vi "GarageDoorOpenCommand_Create.vi"(8 "error in":errorcluster, 10 "GarageDoor":refnum<class "GarageDoor.lvclass">, 11 "reference in":refnum<class "GarageDoorOpenCommand.lvclass">) -> (0 "error out":errorcluster, 3 "reference out":refnum<class "GarageDoorOpenCommand.lvclass">)   [LabVIEW 2020, in "GarageDoorOpenCommand.lvclass"]
uses:
  GarageDoorOpenCommand.lvclass
  C:/Projects/OpenGDS_DesignPatterns/Command1/Command_class/Command.lvclass
  GarageDoor_class/GarageDoor.lvclass
  Command_class/Command.lvclass
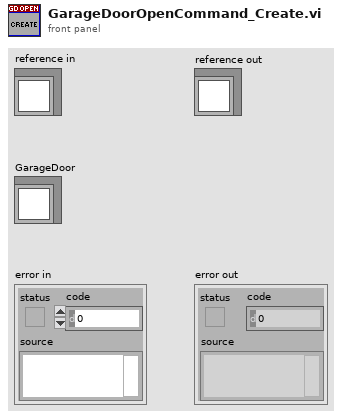
[diagram p1: front panel]
types:
  T1 = typedef "GarageDoorOpenCommand.lvclass/ObjectAttributes.ctl" = cluster{"GarageDoor":refnum<class "GarageDoor.lvclass">}
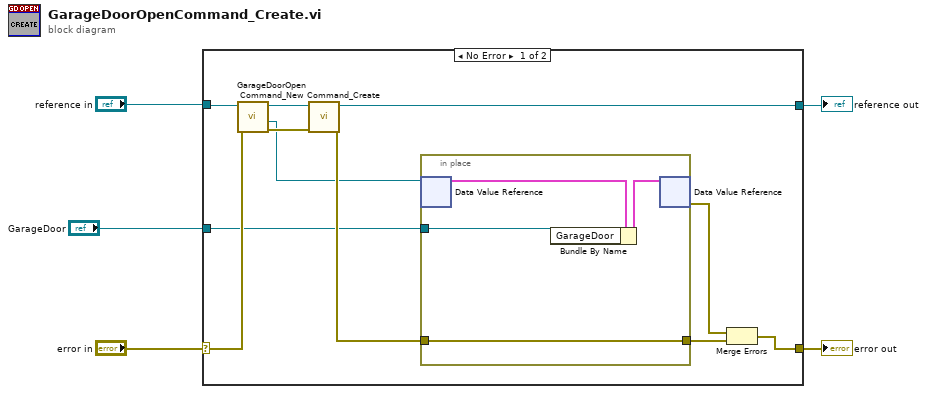
[diagram p0: block diagram]
diagram:
  n1 = case shown="No Error" "error in" {
    selector: "error in" -> [w15 w22]
    tunnel: [w13 w22] -> w4
    tunnel: "reference in" -> [w9 w21]
    tunnel: [w8 w21] -> w2
    tunnel: "GarageDoor" -> [w6 _]
    frame No Error {
      n2 = call "GarageDoorOpenCommand_New.vi"("error in (no error)"=w15, "reference in"=w9) -> ("error out"=w16:errorcluster, "DVRRefOut"=w7:refnum<data-value>, "reference out"=w10:refnum<class "GarageDoorOpenCommand.lvclass">)  [unwired: 6 in, 1 out]
      n3 = call "Command_Create.vi"("error in (no error)"=w16, "reference in"=w10) -> ("error out"=w12:errorcluster, "reference out"=w8:refnum<class "GarageDoorOpenCommand.lvclass">)  [unwired: 8 in]
      n4 = in-place {
        in-place-border: w12 -> [w20]
        in-place-border: [w20] -> w11
        in-place-border: w6 -> [w17]
        n5 = in-place-dvr #1(w7) -> (w18:T1)  [unwired: 1 out]
        n6 = Bundle By Name(cluster=w18, "GarageDoor"=w17) -> (w19:T1)
        n7 = in-place-dvr #1(w19) -> (w14:errorcluster)  [unwired: 1 out]
      }
      n8 = Merge Errors(w14, w11) -> (w13:errorcluster)
    }
    frame Error {
    }
  }
  "error out" <- w4
  "reference out" <- w2
